vi "CST_1298RShadowRegister.VI"() -> (1 "DUTRegisters":T2={"ID"={"REV_ID"=0, "DEV_ID"=enum."ADS1294"}, "Config1 "={"HR"=enum."Low Power Mode", "DAISY_EN"=enum."Daisy Chain Mode", "CLK_EN"=enum."Output Disabled", "DR"=enum."f(MOD) /16"}, "Config2 "={"INT_TEST"=enum."Driven Externally", "TEST_AMP"=enum."(VREFP-VREFN)/2.4", "TEST_FREQ"=enum."f(CLK)/2^21"}, "Config3 "={"PD_REFBUF"=enum."Powered down", "VREFP"=enum."VREFP = 2.4V", "RLD_MEAS"=enum."Open", "RLDREF_INT"=enum."RLDREF fed externally", "PD_RLD"=enum."Powered down"}, "Config4"={"RESP_FREQ"=enum."64kHz", "PULSE_MODE"=enum."Disable", "PDB_LOFF_COMP"=enum."Disable"}, "CH1SET"={"PD"=enum."Normal Operation", "GAIN"=enum."6", "MUXn"=enum."Normal Electrode"}, "CH2SET"={"PD"=enum."Normal Operation", "GAIN"=enum."6", "MUXn"=enum."Normal Electrode"}, "CH3SET"={"PD"=enum."Normal Operation", "GAIN"=enum."6", "MUXn"=enum."Normal Electrode"}, "CH4SET"={"PD"=enum."Normal Operation", "GAIN"=enum."6", "MUXn"=enum."Normal Electrode"}, "CH5SET"={"PD"=enum."Normal Operation", "GAIN"=enum."6", "MUXn"=enum."Normal Electrode"}, "CH6SET"={"PD"=enum."Normal Operation", "GAIN"=enum."6", "MUXn"=enum."Normal Electrode"}, "CH7SET"={"PD"=enum."Power-down", "GAIN"=enum."6", "MUXn"=enum."Normal Electrode"}, "CH8SET"={"PD"=enum."Normal Operation", "GAIN"=enum."6", "MUXn"=enum."Normal Electrode"}, "RESP"={"RESP_DEMOD_EN1"=enum."Disable", "RESP_MOD_EN1"=enum."Disable", "RESP_MOD_VREFP"=enum."VREFP", "RESP_PH"=enum."22.5 deg", "RESP_CTRL"=enum."Mode Disabled"}, "PACE"={"PACEE"=enum."CH2", "PACEO"=enum."CH1", "PDB_PACE"=enum."Buffer Off"}, "LOFF "={"COMP_TH"=enum."Positive - 90% : Negative - 10%", "VLEAD_OFF_EN"=enum."Current Mode", "ILEAD_OFF"=enum."12nA", "FLEAD_OFF"=enum."AC Lead-off Detection at f(DR)/4"}, "WCT1"={"aVF_CH6"=enum."Disable", "aVL_CH5"=enum."Disable", "aVR_CH7"=enum."Enable", "aVR_CH4"=enum."Disable", "PDB_WCTA"=enum."Powered down", "WCTA"=enum."CH1 Positive Input"}, "WCT2"={"PDB_WCTB"=enum."Powered down", "PDB_WCTC"=enum."Powered down", "WCTB"=enum."CH1 Negative Input", "WCTC"=enum."CH1 Positive Input"}, "RLD_SENSP"=[], "RLD_SENSN"=[], "LOFF_STATP"=[], "LOFF_STATN"=[], "LOFF_SENSP"=[], "LOFF_SENSN"=[], "LOFF_FLIP"=[], "GPIO"={"Data"=[], "Direction"=[]}}, 2 "ShadowReg Reg Refs":T1)   [LabVIEW 2010]
doc: "This VI is a constant for the shadow register to store values during app.\n\nInputs:\n<None>\n\nOutputs:\nDUTRegisters (typedef of cooresponding control)\nShadowReg Reg Refs - (cluster[]) names and references to the controls in the shadow register. Allows for searching and indexing."
uses:
  Controls/Shift Registers/TYP_1298RShadowRegister.ctl
  Controls/Register/TYP_Reg_ID.ctl
  Controls/Register/TYP_Reg_CONFIG1.ctl
  Controls/Register/TYP_Reg_CONFIG2.ctl
  Controls/Register/TYP_Reg_CONFIG3.ctl
  Controls/Register/TYP_Reg_CONFIG4.ctl
  Controls/Register/TYP_Reg_CHxSET.ctl
  Controls/Register/TYP_Reg_1298R_RESP.ctl
  Controls/Register/TYP_Reg_PACE.ctl
  Controls/Register/TYP_Reg_LOFF.ctl
  Controls/Register/TYP_Reg_WCT1.ctl
  Controls/Register/TYP_Reg_WCT2.ctl
  Controls/Shift Registers/TYP_CtrlNameArray.ctl
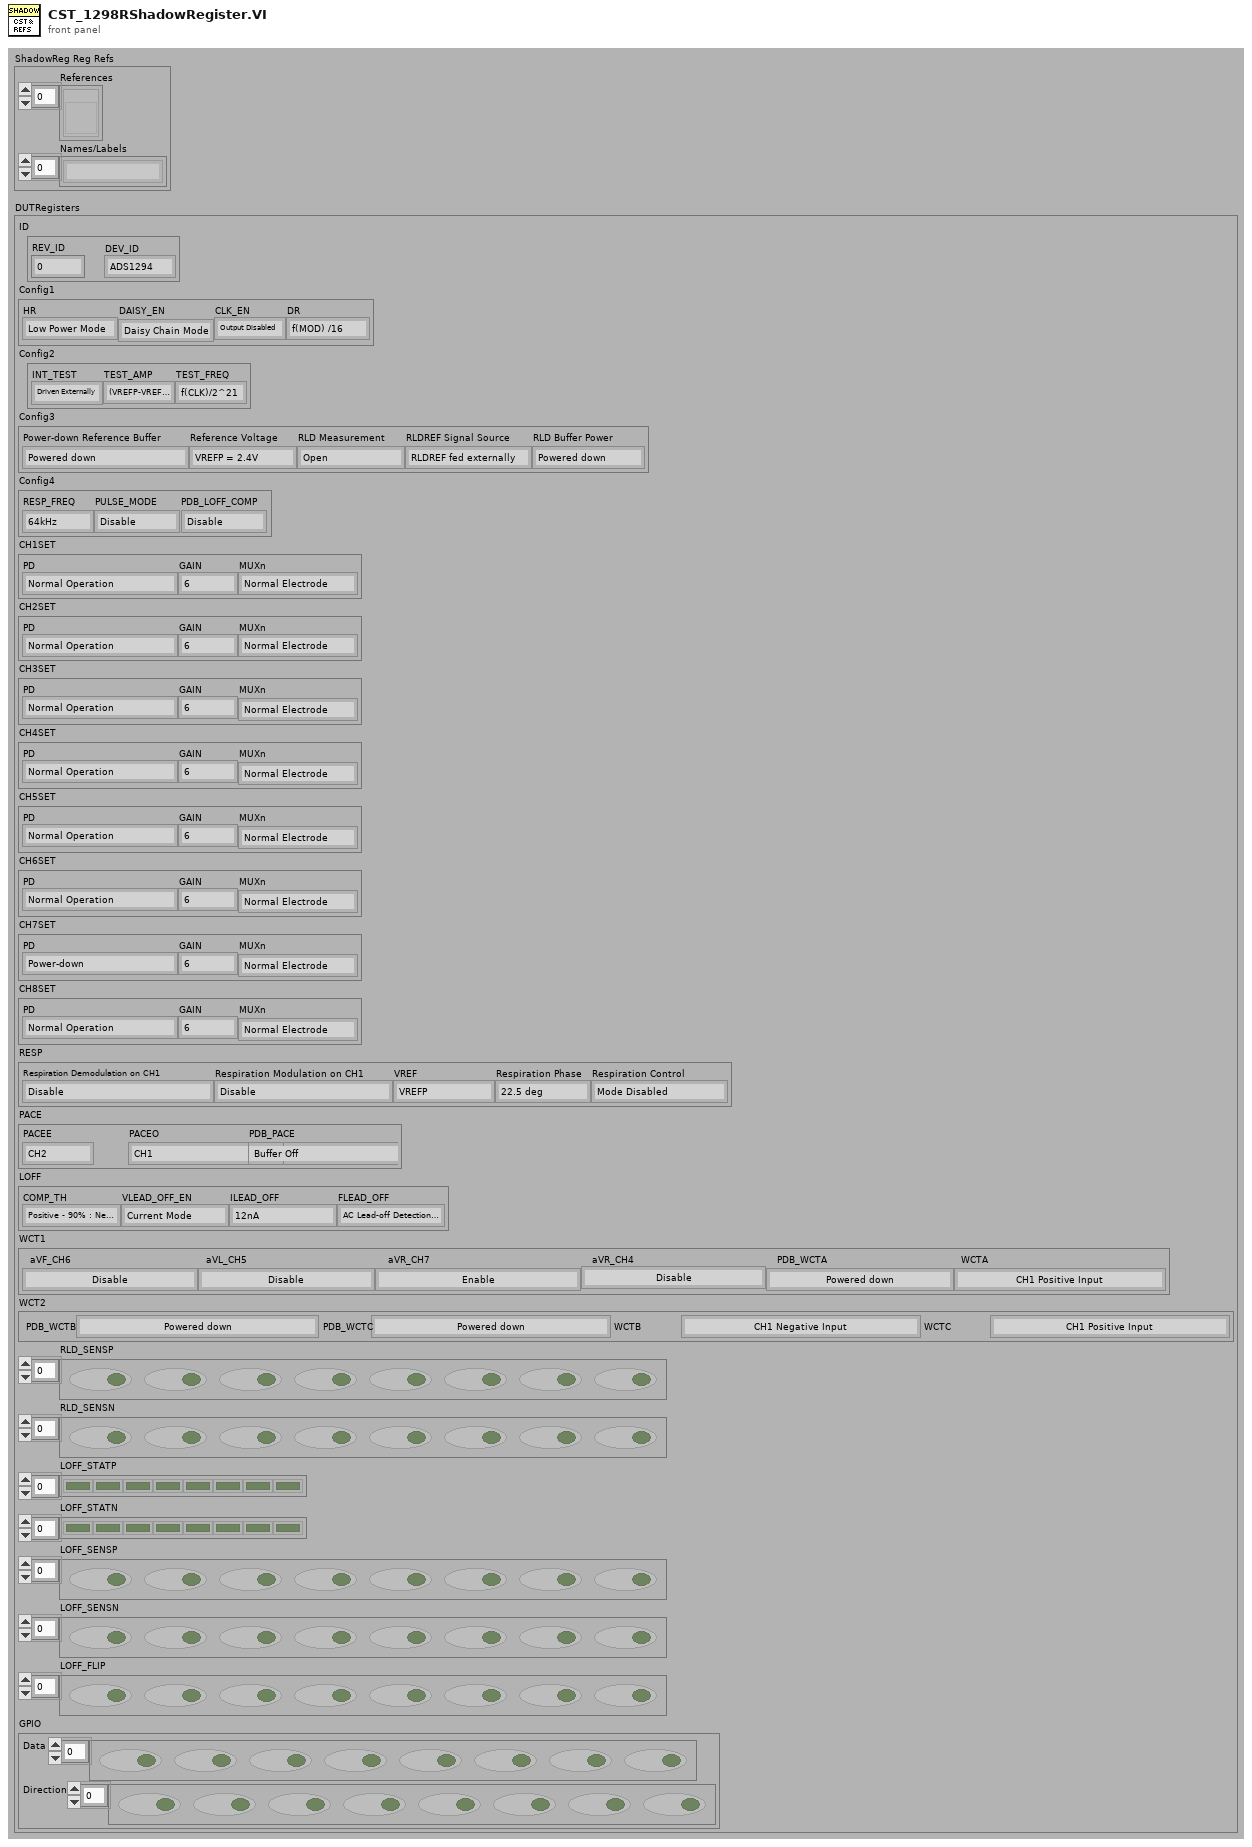
[diagram p1: front panel]
types:
  T1 = typedef "TYP_CtrlNameArray.ctl" = cluster{"References":refnum<vi>[], "Names/Labels":string[]}
  T2 = typedef "TYP_1298RShadowRegister.ctl" = cluster{"ID":T3, "Config1 ":T4, "Config2 ":T5, "Config3 ":T6, "Config4":T7, "CH1SET":T8, "CH2SET":T8, "CH3SET":T8, "CH4SET":T8, "CH5SET":T8, "CH6SET":T8, "CH7SET":T8, "CH8SET":T8, "RESP":T9, "PACE":T10, "LOFF ":T11, "WCT1":T12, "WCT2":T13, "RLD_SENSP":bool[], "RLD_SENSN":bool[], "LOFF_STATP":bool[], "LOFF_STATN":bool[], "LOFF_SENSP":bool[], "LOFF_SENSN":bool[], "LOFF_FLIP":bool[], "GPIO":cluster{"Data":bool[], "Direction":bool[]}}
  T3 = typedef "TYP_Reg_ID.ctl" = cluster{"REV_ID":u8, "DEV_ID":enum8{"ADS1294", "ADS1296", "ADS1298", "N/A", "ADS1194", "ADS1196", "ADS1198"}}
  T4 = typedef "TYP_Reg_CONFIG1.ctl" = cluster{"HR":enum16{"Low Power Mode", "High Resolution Mode"}, "DAISY_EN":enum16{"Daisy Chain Mode", "Multiple Readback Mode"}, "CLK_EN":enum16{"Output Disabled", "Output Enabled"}, "DR":enum16{"f(MOD) /16", "f(MOD) /32", "f(MOD) /64", "f(MOD) /128", "f(MOD) /256", "f(MOD) /512", "f(MOD) /1024"}}
  T5 = typedef "TYP_Reg_CONFIG2.ctl" = cluster{"INT_TEST":enum16{"Driven Externally", "Generated Internally"}, "TEST_AMP":enum16{"(VREFP-VREFN)/2.4", "2x(VREFP-VREFN)/2.4"}, "TEST_FREQ":enum16{"f(CLK)/2^21", "f(CLK)/2^20", "N/A", "DC"}}
  T6 = typedef "TYP_Reg_CONFIG3.ctl" = cluster{"PD_REFBUF":enum16{"Powered down", "Enabled"}, "VREFP":enum16{"VREFP = 2.4V", "VREFP = 4V"}, "RLD_MEAS":enum16{"Open", "RLD_IN Routed"}, "RLDREF_INT":enum16{"RLDREF fed externally", "RLDREF = AVDD/2"}, "PD_RLD":enum16{"Powered down", "Enabled"}}
  T7 = typedef "TYP_Reg_CONFIG4.ctl" = cluster{"RESP_FREQ":enum16{"64kHz", "32kHz", "16kHz", "8kHz", "4kHz", "2kHz", "1kHz", "500Hz"}, "PULSE_MODE":enum16{"Disable", "Enable"}, "PDB_LOFF_COMP":enum16{"Disable", "Enable"}}
  T8 = typedef "TYP_Reg_CHxSET.ctl" = cluster{"PD":enum16{"Normal Operation", "Power-down"}, "GAIN":enum16{"6", "1", "2", "3", "4", "8", "12"}, "MUXn":enum16{"Normal Electrode", "Input Short", "RLD Measurement", "MVDD", "Temperature Sensor", "Test Signal", "RLD Positive Electrode Driver", "RLD Negative electrode Driver"}}
  T9 = typedef "TYP_Reg_1298R_RESP.ctl" = cluster{"RESP_DEMOD_EN1":enum16{"Disable", "Enable"}, "RESP_MOD_EN1":enum16{"Disable", "Enable"}, "RESP_MOD_VREFP":enum16{"AVDD", "VREFP"}, "RESP_PH":enum16{"22.5 deg", "45 deg", "67.5 deg", "90 deg", "112.5 deg", "135 deg", "157.5 deg", "180 deg"}, "RESP_CTRL":enum16{"Mode Disabled", "External Respiration", "Int. Resp. with Int. CLK", "Int. Resp. with Ext. CLK"}}
  T10 = typedef "TYP_Reg_PACE.ctl" = cluster{"PACEE":enum16{"CH2", "CH4", "CH6", "CH8"}, "PACEO":enum16{"CH1", "CH3", "CH5", "CH7"}, "PDB_PACE":enum16{"Buffer Off", "Buffer On"}}
  T11 = typedef "TYP_Reg_LOFF.ctl" = cluster{"COMP_TH":enum16{"Positive - 95% : Negative - 5%", "Positive - 92.5% : Negative - 7.5%", "Positive - 90% : Negative - 10%", "Positive - 87.5% : Negative - 12.5%", "Positive - 85% : Negative - 15%", "Positive - 80% : Negative - 20%", "Positive - 75% : Negative - 25%", "Positive - 70% : Negative - 30%"}, "VLEAD_OFF_EN":enum16{"Current Mode", "Pull-up/Pull-Down Resistor Mode"}, "ILEAD_OFF":enum16{"6nA", "12nA", "18nA", "24nA"}, "FLEAD_OFF":enum16{"Disabled", "AC Lead-off Detection at f(DR)/4", "N/A", "DC Lead-off Detection ON"}}
  T12 = typedef "TYP_Reg_WCT1.ctl" = cluster{"aVF_CH6":enum16{"Disable", "Enable"}, "aVL_CH5":enum16{"Disable", "Enable"}, "aVR_CH7":enum16{"Disable", "Enable"}, "aVR_CH4":enum16{"Disable", "Enable"}, "PDB_WCTA":enum16{"Powered down", "Powered on"}, "WCTA":enum16{"CH1 Positive Input", "CH1 Negative Input", "CH2 Positive Input", "CH2 Negative Input", "CH3 Positive Input", "CH3 Negative Input", "CH4 Positive Input", "CH4 Negative Input"}}
  T13 = typedef "TYP_Reg_WCT2.ctl" = cluster{"PDB_WCTB":enum16{"Powered down", "Powered on"}, "PDB_WCTC":enum16{"Powered down", "Powered on"}, "WCTB":enum16{"CH1 Positive Input", "CH1 Negative Input", "CH2 Positive Input", "CH2 Negative Input", "CH3 Positive Input", "CH3 Negative Input", "CH4 Positive Input", "CH4 Negative Input"}, "WCTC":enum16{"CH1 Positive Input", "CH1 Negative Input", "CH2 Positive Input", "CH2 Negative Input", "CH3 Positive Input", "CH3 Negative Input", "CH4 Positive Input", "CH4 Negative Input"}}
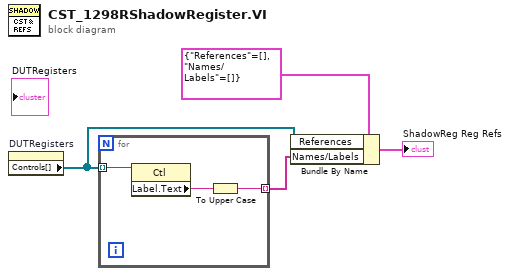
[diagram p0: block diagram]
diagram:
  n1 = property on="DUTRegisters" class="Clust (strict)"() -> ("Controls[]"=w4:refnum<vi>[])  [unwired: 2 in, 2 out]
  n2 = for {
    tunnel: w4 -> [w7] mode=indexing
    tunnel: [w5] -> w3 mode=indexing
    n3 = property class="Ctl"(reference=w7) -> ("Label.Text"=w6:string)  [unwired: 1 in, 2 out]
    n4 = To Upper Case(1:w6) -> (0:w5:string)
  }
  n5 = Bundle By Name(cluster=T1 {"References"=[], "Names/Labels"=[]} ("ControlRef Array"), "References"=w4, "Names/Labels"=w3) -> (→"ShadowReg Reg Refs":T1)
